vi "OldClimbSetSensorPoseLeft.vi"(8 "ClimbSetSensorPoseLeft":dbl) -> ()   [LabVIEW 2023]
uses:
  OldClimbGlobal.vi
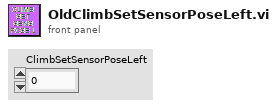
[diagram p1: front panel]
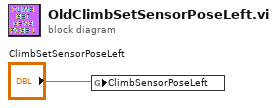
[diagram p0: block diagram]
diagram:
  n1 = global write "OldClimbGlobal.vi" "ClimbSensorPoseLeft"("ClimbSetSensorPoseLeft") -> ()
